vi "Add Plugin with Children.vi"(8 "error in (no error)":errorcluster, 9 "Plugin":refnum<class "Plugin.lvclass">, 10 "parent tag":string, 11 "Application Data In":T1) -> (0 "error out":errorcluster, 3 "Application Data Out":T1)   [LabVIEW 2017, in "DSF Data Viewer.lvlib"]
uses:
  DSF Data Viewer.lvlib
  Main VI/Application Data.ctl
  <vilib>/NI/Memory Manager/Classes/Pointer/Pointer.lvclass
  Builds/Data Sharing Framework/Current/Core/DSF Core.lvlibp/Engine/Classes/Framework/Framework.lvclass
  Buffer Reader/Buffer Data.ctl
  Builds/Data Sharing Framework/Current/Core/DSF Core.lvlibp/Engine/Classes/Buffer/Buffer.lvclass
  Builds/Data Sharing Framework/Current/Core/DSF Core.lvlibp/Engine/Classes/Transfer Group Status/Transfer Group Status.lvclass
  Builds/Data Sharing Framework/Current/Core/DSF Core.lvlibp/Engine/Classes/Plugin/Plugin.lvclass
  ID to Tree Items/Tree Item Type.ctl
  Add Transfer.vi
  Add Buffers.vi
  Builds/Data Sharing Framework/Current/Core/DSF Core.lvlibp/Engine/Classes/Buffer/Get Async Buffer.vi
  Builds/Data Sharing Framework/Current/Core/DSF Core.lvlibp/Engine/Classes/Buffer/Get Inline Buffer.vi
  Builds/Data Sharing Framework/Current/Core/DSF Core.lvlibp/Engine/Classes/Transfer Group/Get Inline.vi
  Builds/Data Sharing Framework/Current/Core/DSF Core.lvlibp/Engine/Classes/Transfer Group/Get Transfers.vi
  Builds/Data Sharing Framework/Current/Core/DSF Core.lvlibp/Engine/Classes/Transfer Group/Get Status.vi
  Builds/Data Sharing Framework/Current/Core/DSF Core.lvlibp/Engine/Classes/Timing/Timing.lvclass
  Builds/Data Sharing Framework/Current/Core/DSF Core.lvlibp/Engine/Classes/Buffer/Buffers.lvclass
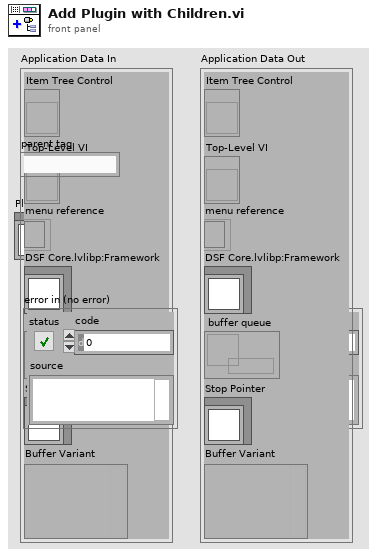
[diagram p1: front panel]
types:
  T1 = typedef "DSF Data Viewer.lvlib/Application Data.ctl" = cluster{"Item Tree Control":refnum<vi>, "Top-Level VI":refnum<vi>, "menu reference":refnum<k9>, "DSF Core.lvlibp:Framework":refnum<class "Framework.lvclass">, "buffer queue":refnum<queue>, "Stop Pointer":refnum<class "Pointer.lvclass">, "Buffer Variant":variant}
  T2 = typedef "DSF Data Viewer.lvlib/Buffer Data.ctl" = cluster{"DSF Core.lvlibp:Buffer":refnum<class "Buffer.lvclass">, "DSF Core.lvlibp:Transfer Group Status.lvclass":refnum<class "Transfer Group Status.lvclass">, "decimation":u64}
  T3 = typedef "DSF Data Viewer.lvlib/Tree Item Type.ctl" = enum16{"Framework", "Plugin Group", "Plugin", "Group", "Transfer", "Buffer", "Channel"}
  T4 = typedef "DSF Data Viewer.lvlib/Tree Item.ctl" = cluster{"Left Cell String":string, "Child Text":string[], "Child Tag":string, "Glyph Index":i32}
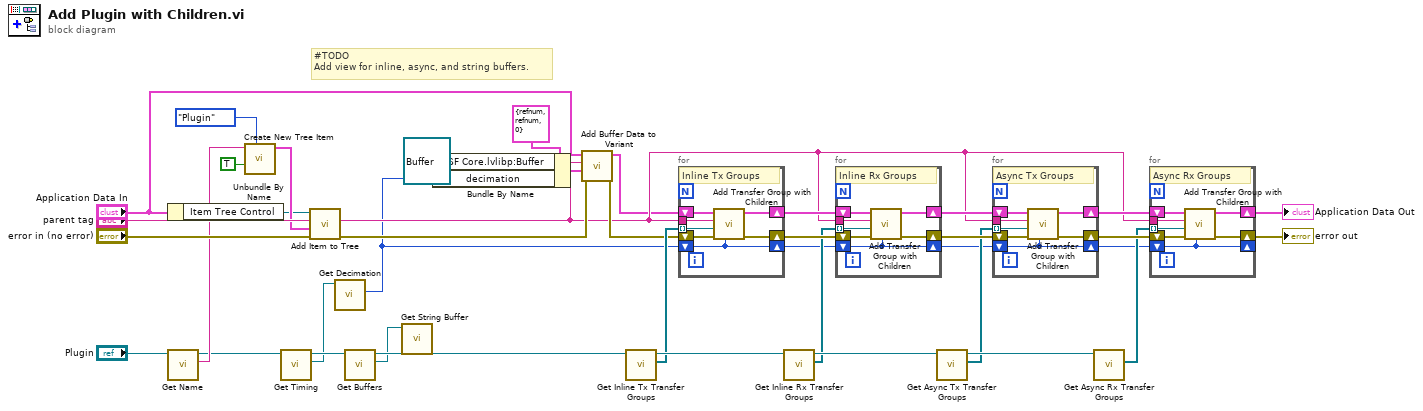
[diagram p0: block diagram]
diagram:
  # "#TODO\nAdd view for inline, async, and string buffers."
  n1 = Unbundle By Name("Application Data In") -> ("Item Tree Control"=w19:refnum<vi>)
  n2 = call "Get Name.vi"("Plugin in"="Plugin") -> ("name"=w31:string)  [unwired: 9 in, 1 out]
  n3 = call "Create New Tree Item.vi"("Item Type"=Tree_Item_Type."Plugin", "found?"=TRUE, "Left Cell String"=w31) -> ("Item"=w32:T4)  [unwired: 7 in, 1 out]
  n4 = call "Get Timing.vi"("Plugin in"="Plugin") -> ("Timing"=w9:refnum<class "Timing.lvclass">, "Plugin out"=w11:refnum<class "Plugin.lvclass">)  [unwired: 9 in]
  n5 = call "Add Item to Tree.vi"("error in (no error)"="error in (no error)", "Item"=w32, "parent tag"="parent tag", "TreeControl in"=w19) -> ("error out"=w18:errorcluster, "new item tag"=w12:string)  [unwired: 5 in, 1 out]
  n6 = call "Get Decimation.vi"("Timing in"=w9) -> ("Decimation"=w5:u64)  [unwired: 9 in, 1 out]
  n7 = call "Get Buffers.vi"("Plugin in"=w11) -> ("Buffers"=w8:refnum<class "Buffers.lvclass">, "Plugin out"=w10:refnum<class "Plugin.lvclass">)  [unwired: 9 in]
  n8 = call "Get String Buffer.vi"("Buffers in"=w8) -> ()  [unwired: 9 in, 2 out]
  n9 = Bundle By Name(cluster=T2 {"DSF Core.lvlibp:Buffer"=refnum, "DSF Core.lvlibp:Transfer Group Status.lvclass"=refnum, "decimation"=0} ("Buffer data"), "DSF Core.lvlibp:Buffer"=refnum<class "Buffer.lvclass"> refnum ("Buffer"), "decimation"=w5) -> (w13:T2)
  n10 = call "Add Buffer Data to Variant.vi"("error in (no error)"=w18, "Buffer data"=w13, "tag"=w12, "Application Data In in"="Application Data In") -> ("error out"=w16:errorcluster, "Application Data In out"=w7:T1)  [unwired: 6 in]
  n11 = call "Get Inline Tx Transfer Groups.vi"("Plugin in"=w10) -> ("Inline Tx Transfer Groups"=w30:refnum<class "Transfer Group.lvclass">[], "Plugin out"=w35:refnum<class "Plugin.lvclass">)  [unwired: 9 in]
  n12 = for {
    tunnel: w12 -> [w41]
    tunnel: w30 -> [w42] mode=indexing
    shift-right: [w43] -> w29
    shift-left: w7 -> [w46]
    shift-right: [w44] -> w28
    shift-left: w16 -> [w45]
    shift-right: [w40] -> w4
    shift-left: w5 -> [w40]
    # "Inline Tx Groups"
    n13 = call "Add Transfer Group with Children.vi"("Plugin Decimation (1)"=w40, "error in (no error)"=w45, "Transfer Group"=w42, "parent tag"=w41, "Application Data In"=w46) -> ("error out"=w44:errorcluster, "Application Data In"=w43:T1)  [unwired: 5 in]
  }
  n14 = call "Get Inline Rx Transfer Groups.vi"("Plugin in"=w35) -> ("Inline Rx Transfer Groups"=w23:refnum<class "Transfer Group.lvclass">[], "Plugin out"=w34:refnum<class "Plugin.lvclass">)  [unwired: 9 in]
  n15 = for {
    tunnel: w12 -> [w48]
    tunnel: w23 -> [w49] mode=indexing
    shift-right: [w50] -> w27
    shift-left: w29 -> [w53]
    shift-right: [w51] -> w26
    shift-left: w28 -> [w52]
    shift-right: [w47] -> w3
    shift-left: w4 -> [w47]
    # "Inline Rx Groups"
    n16 = call "Add Transfer Group with Children.vi"("Plugin Decimation (1)"=w47, "error in (no error)"=w52, "Transfer Group"=w49, "parent tag"=w48, "Application Data In"=w53) -> ("error out"=w51:errorcluster, "Application Data In"=w50:T1)  [unwired: 5 in]
  }
  n17 = call "Get Async Tx Transfer Groups.vi"("Plugin in"=w34) -> ("Async Tx Transfer Groups"=w22:refnum<class "Transfer Group.lvclass">[], "Plugin out"=w33:refnum<class "Plugin.lvclass">)  [unwired: 9 in]
  n18 = for {
    tunnel: w12 -> [w55]
    tunnel: w22 -> [w56] mode=indexing
    shift-right: [w57] -> w25
    shift-left: w27 -> [w60]
    shift-right: [w58] -> w24
    shift-left: w26 -> [w59]
    shift-right: [w54] -> w2
    shift-left: w3 -> [w54]
    # "Async Tx Groups"
    n19 = call "Add Transfer Group with Children.vi"("Plugin Decimation (1)"=w54, "error in (no error)"=w59, "Transfer Group"=w56, "parent tag"=w55, "Application Data In"=w60) -> ("error out"=w58:errorcluster, "Application Data In"=w57:T1)  [unwired: 5 in]
  }
  n20 = call "Get Async Rx Transfer Groups.vi"("Plugin in"=w33) -> ("Async Rx Transfer Groups"=w21:refnum<class "Transfer Group.lvclass">[])  [unwired: 9 in, 1 out]
  n21 = for {
    tunnel: w12 -> [w62]
    tunnel: w21 -> [w63] mode=indexing
    shift-right: [w64] -> w6
    shift-left: w25 -> [w67]
    shift-right: [w65] -> w20
    shift-left: w24 -> [w66]
    shift-right: [w61] -> _
    shift-left: w2 -> [w61]
    # "Async Rx Groups"
    n22 = call "Add Transfer Group with Children.vi"("Plugin Decimation (1)"=w61, "error in (no error)"=w66, "Transfer Group"=w63, "parent tag"=w62, "Application Data In"=w67) -> ("error out"=w65:errorcluster, "Application Data In"=w64:T1)  [unwired: 5 in]
  }
  "error out" <- w20
  "Application Data Out" <- w6
